vi "CAN_GetReceiveNum.vi"(8 "错误输入（无错误） 2":errorcluster caption="错误输入（无错误）", 11 "General_Input":T1={"DevType"=1, "DevIndex"=0, "CANIndex"=0} {"CANIndex" items=["0", "1"]; "DevType" items=["PCI5121"=1, "PCI9810"=2, "USBCAN1"=3, "USBCAN2"=4, "PCI9820"=5, "CAN232"=6, "PCI5110"=7, "CANLite(mini)"=8, "ISA9620"=9, "ISA5420"=10, "PC104CAN"=11, "CANETE"=12, "DNP9810"=13, "PCI9840B"=14, "PC104C2"=15, "PCI9820I"=16]}) -> (0 "错误输出":errorcluster, 2 "GetReceiveNum":u32, 3 "General_Output":T1={"DevType"=1, "DevIndex"=0, "CANIndex"=0} {"CANIndex" items=["0", "1"]; "DevType" items=["PCI5121"=1, "PCI9810"=2, "USBCAN1"=3, "USBCAN2"=4, "PCI9820"=5, "CAN232"=6, "PCI5110"=7, "CANLite(mini)"=8, "ISA9620"=9, "ISA5420"=10, "PC104CAN"=11, "CANETE"=12, "DNP9810"=13, "PCI9840B"=14, "PC104C2"=15, "PCI9820I"=16]})   [LabVIEW 2012]
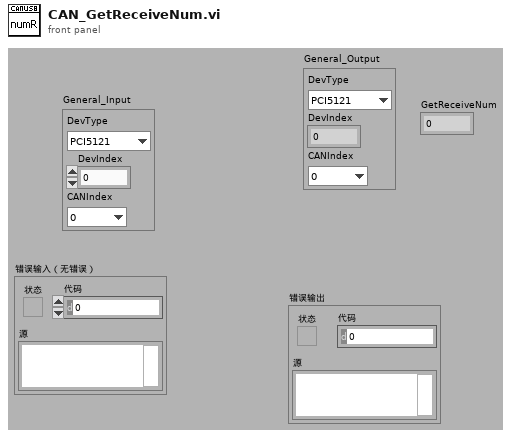
[diagram p1: front panel]
types:
  T1 = cluster{"DevType":u16, "DevIndex":u32, "CANIndex":u16}
  T2 = cluster{"DevType":u32, "DevIndex":u32, "CANIndex":u32}
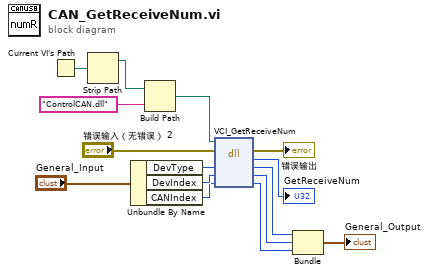
[diagram p0: block diagram]
diagram:
  n1 = Current VI's Path() -> (path=w12:path)
  n2 = Strip Path(path=w12) -> (stripped path=w10:path)  [unwired: 1 out]
  n3 = Unbundle By Name("General_Input") -> ("DevType"=w7:u16, "DevIndex"=w6:u32, "CANIndex"=w5:u16)
  n4 = Build Path(base path=w10, name or relative path="ControlCAN.dll" ("名称或相对路径")) -> (appended path=w9:path)
  n5 = dll-call lib="E:/1_Projects/ITMS/API Library/ControlCAN.dll" fn="VCI_GetReceiveNum"(path in=w9, error in="错误输入（无错误） 2", "DevType"=w7, "DevIndex"=w6, "CANIndex"=w5) -> (error out=→"错误输出":errorcluster, "GetReceiveNum"=→"GetReceiveNum":u32, "DevType"=w4:u32, "DevIndex"=w3:u32, "CANIndex"=w2:u32)  [unwired: 1 in, 1 out]
  n6 = Bundle("DevType"=w4, "DevIndex"=w3, "CANIndex"=w2) -> (→"General_Output":T2)  [unwired: 1 in]
